vi "Fdx Get Tx UDP Session Status.vi"(8 "error in (no error)":errorcluster, 10 "UdpHandle in":u32, 11 "InstrumentHandle_port in":u32) -> (0 "error out":errorcluster, 1 "CurrentIndex":u32, 2 "UdpHandle out":u32, 3 "InstrumentHandle_port out":u32, 4 "IndexCycleCount":u32, 5 "MsgCount":u32)   [LabVIEW 2020, in "AIM664LV.lvlib"]
uses:
  AIM664LV.lvlib
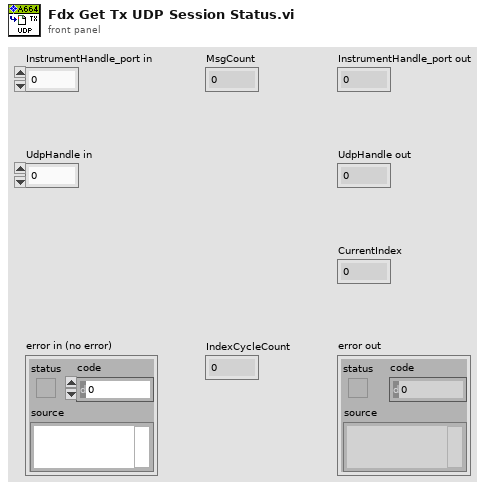
[diagram p1: front panel]
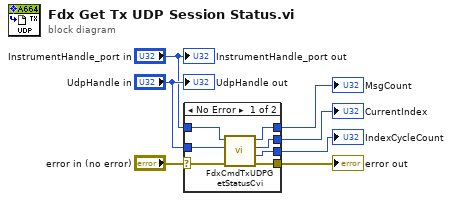
[diagram p0: block diagram]
diagram:
  n1 = case shown="No Error" "error in (no error)" {
    selector: "error in (no error)" -> [w14 w15]
    tunnel: [w13 w15] -> w6
    tunnel: [w12 _] -> w5
    tunnel: [w11 _] -> w4
    tunnel: [w10 _] -> w3
    tunnel: "UdpHandle in" -> [w9 _]
    tunnel: "InstrumentHandle_port in" -> [w8 _]
    frame No Error {
      n2 = call "FdxCmdTxUDPGetStatusCvi.vi"("error in"=w14, "UdpHandle"=w9, "InstrumentHandle"=w8) -> ("error out"=w13:errorcluster, "IndexCycleCount"=w10:u32, "CurrentIndex"=w11:u32, "MsgCount"=w12:u32)  [unwired: 4 in, 1 out]
    }
    frame Error {
    }
  }
  "error out" <- w6
  "MsgCount" <- w5
  "CurrentIndex" <- w4
  "IndexCycleCount" <- w3
  "InstrumentHandle_port out" <- "InstrumentHandle_port in"
  "UdpHandle out" <- "UdpHandle in"
